vi "fitHyperbolamodel.vi"(3 "lambda":dbl=1e-10, 4 "Z":dbl[](array[numeric]), 5 "Wz":dbl[](array[numeric])) -> (0 "最佳拟合":dbl[](array[numeric]), 1 "发散角":dbl)   [LabVIEW 2018]
uses:
  <vilib>/gmath/NumericalOptimization/Nonlinear Curve Fit LM.vi
  <vilib>/gmath/NI_Gmath.lvlib
panel:
  out "参数":dbl
  out "残差最小值":dbl
  out "L0":dbl
  out "XY图":cluster{"Z":dbl[], "f(X,a)":dbl[]}[](graph)
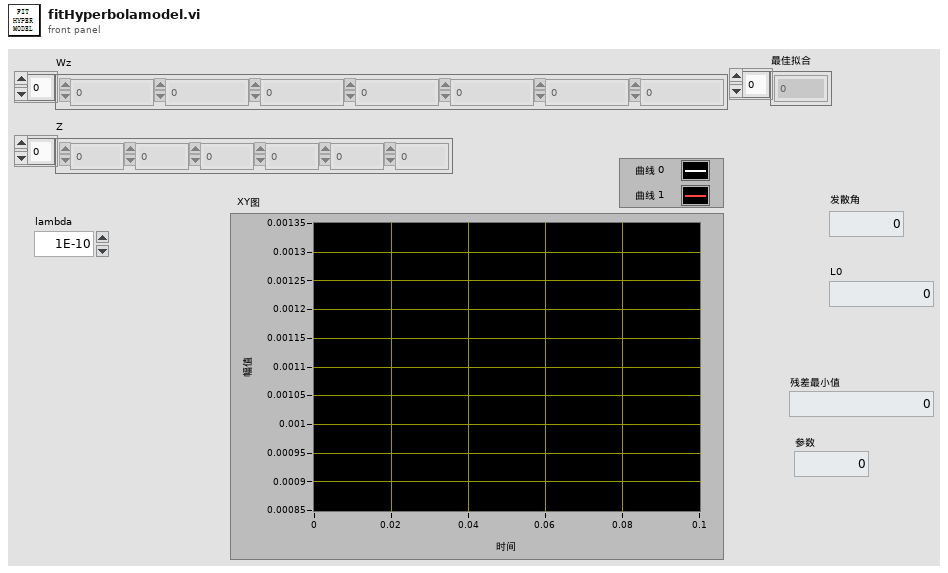
[diagram p1: front panel]
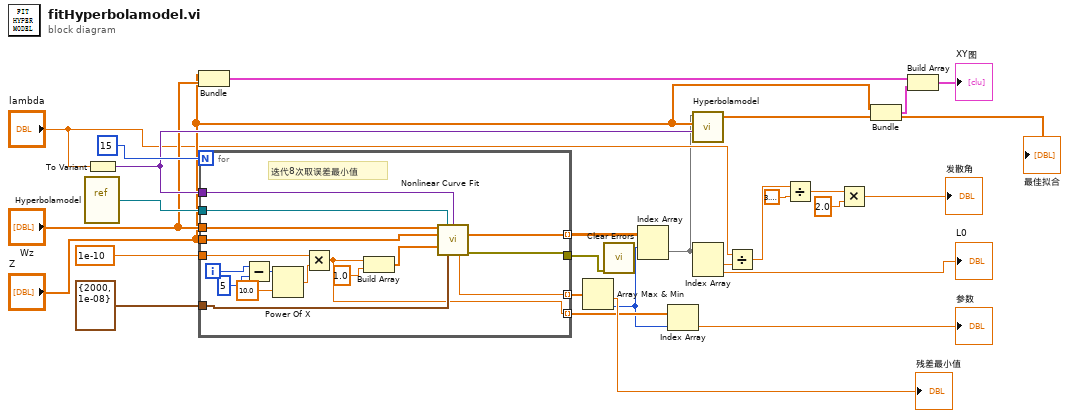
[diagram p0: block diagram]
diagram:
  n1 = vi-ref "Hyperbolamodel.vi"() -> (w25:refnum<vi>)
  n2 = To Variant(anything="lambda") -> (Variant=w23:variant)
  n3 = Bundle("Z"="Z", "Wz"="Wz") -> (w19:cluster{"Z":dbl[], "Wz":dbl[]})  [unwired: 1 in]
  n4 = for {
    N: 15 -> [_]
    tunnel: "Wz" -> [w44]
    tunnel: "Z" -> [w43]
    tunnel: w23 -> [w42]
    tunnel: w25 -> [w41]
    tunnel: cluster{"max iteration":i32, "tolerance":dbl} {"max iteration"=2000, "tolerance"=1e-08} ("termination") -> [w40]
    tunnel: [w37] -> w10 mode=indexing
    tunnel: [w33] -> w5 mode=indexing
    tunnel: 1e-10 -> [w35]
    tunnel: [w32] -> w2 mode=indexing
    tunnel: [w28] -> w1
    i -> [w31]
    # "迭代8次取误差最小值"
    n5 = Subtract(x=w31, y=5) -> (x-y=w29:i32)
    n6 = Power Of X(1:10.0 ("x"), 2:w29) -> (0:w34:dbl)
    n7 = Multiply(x=w35, y=w34) -> (x*y=w33:dbl)
    n8 = Build Array(w33, 1.0 ("元素")) -> (w39:dbl[])
    n9 = call-poly <vilib>:"Nonlinear Curve Fit.vi"("Y"=w44, "f(x,a)"=w41, "data"=w42, "X"=w43, "initial parameters"=w39, "termination"=w40) -> ("best fit parameters"=w37:dbl[], "residue"=w32:dbl, "error out"=w28:errorcluster)  [unwired: 4 in, 3 out]
  }
  n10 = Array Max & Min(array=w2) -> (min value=→"残差最小值":dbl, min index (indices)=w3:i32)  [unwired: 2 out]
  n11 = call <vilib>:"Clear Errors.vi"("error in (no error)"=w1) -> ()  [unwired: 5 in, 2 out]
  n12 = Index Array(array=w10, index (row)=w3) -> (element=w9:dbl[])  [unwired: 1 in]
  n13 = Index Array(array=w5, index=w3) -> (element=→"参数":dbl)
  n14 = call "Hyperbolamodel.vi"("数据"=w23, "Z"="Z", "a"=w9) -> ("f(X,a)"=w20:dbl[])  [unwired: 1 in, 2 out]
  "最佳拟合" <- w20
  n15 = Index Array(array=w9) -> (element #1=w8:dbl, element #2=→"L0":dbl)  [unwired: 2 in]
  n16 = Divide(x="lambda", y=w8) -> (x/y=w15:dbl)
  n17 = Divide(x=w15, y=3.141592653589793) -> (x/y=w13:dbl)
  n18 = Multiply(x=w13, y=2.0) -> (x*y=→"发散角":dbl)
  n19 = Bundle("Z"="Z", "f(X,a)"=w20) -> (w18:cluster{"Z":dbl[], "f(X,a)":dbl[]})  [unwired: 1 in]
  n20 = Build Array(w19, w18) -> (→"XY图":cluster{"Z":dbl[], "f(X,a)":dbl[]}[])
